vi "Initialize.vi"(8 "error in (no error)":errorcluster, 9 "Y (North)":dbl, 10 "X (East)":dbl) -> (0 "error out":errorcluster, 3 "CartesianVector out":refnum<class "CartesianVector.lvclass">)   [LabVIEW 2012, in "CartesianVector.lvclass"]
doc: "Takes in a X (East) and Y(North) coordinate DBL value and bundles them together to create a CartesianVector object."
uses:
  CartesianVector.lvclass
  CartesianVector.lvclass/CartesianVector.ctl
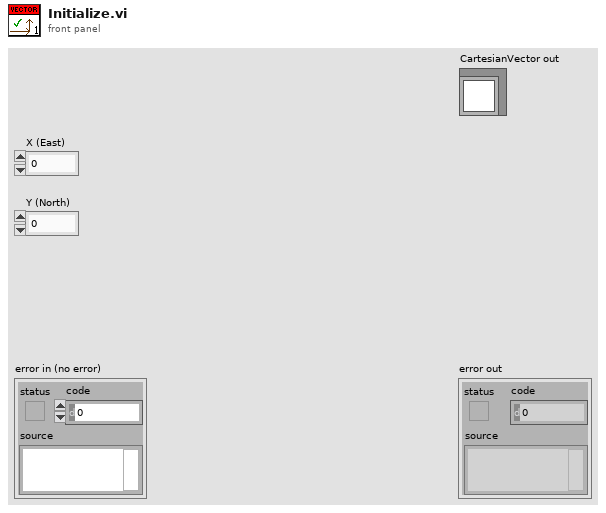
[diagram p1: front panel]
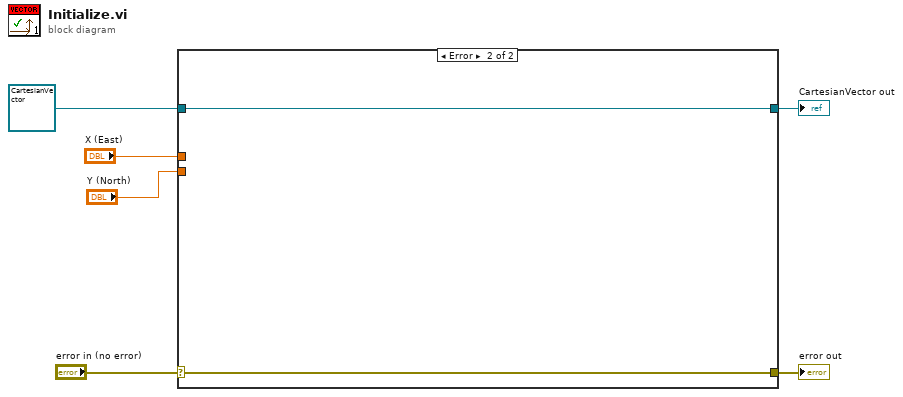
[diagram p0: block diagram]
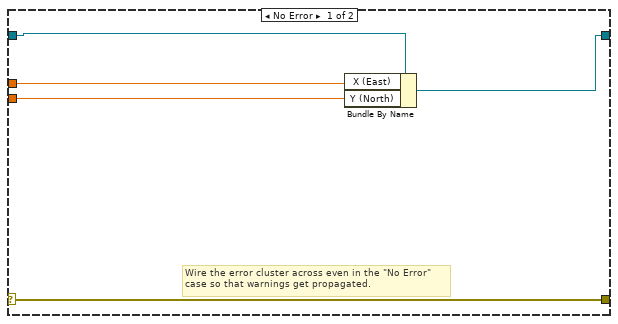
[diagram p2: hidden frame]
diagram:
  n1 = case shown="Error" "error in (no error)" {
    selector: "error in (no error)" -> [w11 w13]
    tunnel: [w11 w13] -> w5
    tunnel: [w7 w12] -> w3
    tunnel: refnum<class "CartesianVector.lvclass"> refnum ("CartesianVector in") -> [w10 w12]
    tunnel: "X (East)" -> [w9 _]
    tunnel: "Y (North)" -> [w8 _]
    frame No Error {
      # "Wire the error cluster across even in the \"No Error\"\ncase so that warnings get propagated."
      n2 = Bundle By Name(cluster=w10, "X (East)"=w9, "Y (North)"=w8) -> (w7:refnum<class "CartesianVector.lvclass">)
    }
    frame Error {
    }
  }
  "error out" <- w5
  "CartesianVector out" <- w3
